vi "Ejercicio 2.2.vi"() -> ()   [LabVIEW 2021]
panel:
  in  "Numeric":dbl
  out "8 BIt":string
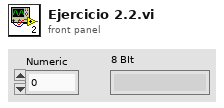
[diagram p1: front panel]
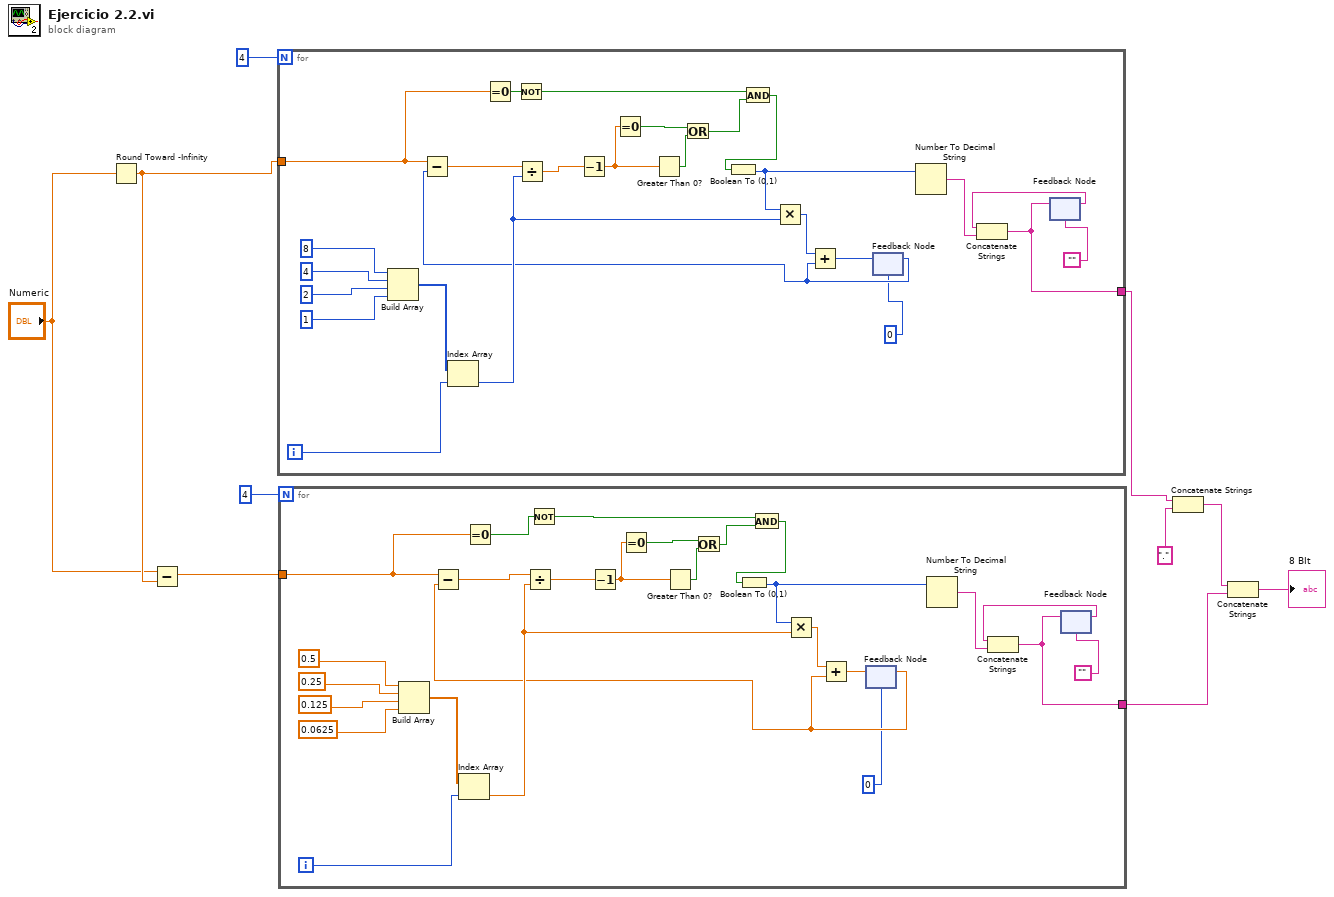
[diagram p0: block diagram]
diagram:
  n1 = Round Toward -Infinity(1:"Numeric") -> (0:w9:dbl)
  n2 = Subtract(x="Numeric", y=w9) -> (x-y=w3:dbl)
  n3 = for {
    N: 4 -> [_]
    tunnel: w9 -> [w20]
    tunnel: [w25] -> w5
    i -> [w31]
    n4 = Build Array(8, 4, 2, 1) -> (w32:i32[])
    n5 = Index Array(array=w32, index=w31) -> (element=w14:i32)
    n6 = Equal To 0?(x=w20) -> (x = 0?=w22:bool)
    n7 = Not(x=w22) -> (.not. x?=w21:bool)
    n8 = feedback #1(0) -> (w12:i32)
    n9 = Subtract(x=w20, y=w12) -> (x-y=w19:dbl)
    n10 = Divide(x=w19, y=w14) -> (x/y=w16:dbl)
    n11 = Decrement(x=w16) -> (x-1=w15:dbl)
    n12 = Equal To 0?(x=w15) -> (x = 0?=w30:bool)
    n13 = Greater Than 0?(x=w15) -> (x > 0?=w29:bool)
    n14 = Or(x=w30, y=w29) -> (x .or. y?=w23:bool)
    n15 = And(x=w21, y=w23) -> (x .and. y?=w17:bool)
    n16 = Boolean To (0,1)(Boolean=w17) -> (0, 1=w18:i16)
    n17 = Multiply(x=w18, y=w14) -> (x*y=w28:i32)
    n18 = Add(x=w28, y=w12) -> (x+y=w13:i32)
    n19 = feedback-in #1(w13) -> ()
    n20 = Number To Decimal String(number=w18) -> (decimal integer string=w27:string)  [unwired: 1 in]
    n21 = feedback #2("") -> (w26:string)
    n22 = Concatenate Strings(w26, w27) -> (w25:string)
    n23 = feedback-in #2(w25) -> ()
  }
  n24 = for {
    N: 4 -> [_]
    tunnel: w3 -> [w40]
    tunnel: [w51] -> w2
    i -> [w61]
    n25 = Build Array(0.5, 0.25, 0.125, 0.0625) -> (w62:dbl[])
    n26 = Index Array(array=w62, index=w61) -> (element=w54:dbl)
    n27 = Equal To 0?(x=w40) -> (x = 0?=w42:bool)
    n28 = Not(x=w42) -> (.not. x?=w41:bool)
    n29 = feedback #3(0) -> (w38:dbl)
    n30 = Subtract(x=w40, y=w38) -> (x-y=w45:dbl)
    n31 = Divide(x=w45, y=w54) -> (x/y=w60:dbl)
    n32 = Decrement(x=w60) -> (x-1=w39:dbl)
    n33 = Equal To 0?(x=w39) -> (x = 0?=w59:bool)
    n34 = Greater Than 0?(x=w39) -> (x > 0?=w58:bool)
    n35 = Or(x=w59, y=w58) -> (x .or. y?=w44:bool)
    n36 = And(x=w41, y=w44) -> (x .and. y?=w43:bool)
    n37 = Boolean To (0,1)(Boolean=w43) -> (0, 1=w57:i16)
    n38 = Multiply(x=w57, y=w54) -> (x*y=w55:dbl)
    n39 = Add(x=w55, y=w38) -> (x+y=w56:dbl)
    n40 = feedback-in #3(w56) -> ()
    n41 = Number To Decimal String(number=w57) -> (decimal integer string=w53:string)  [unwired: 1 in]
    n42 = feedback #4("") -> (w52:string)
    n43 = Concatenate Strings(w52, w53) -> (w51:string)
    n44 = feedback-in #4(w51) -> ()
  }
  n45 = Concatenate Strings(w5, ".") -> (w6:string)
  n46 = Concatenate Strings(w6, w2) -> (→"8 BIt":string)
